vi "start.vi"(8 "error in (no error)":errorcluster, 11 "Pixelfly in":refnum<class "PixelflySA.lvclass">) -> (0 "error out":errorcluster, 3 "Pixelfly out":refnum<class "PixelflySA.lvclass">)   [LabVIEW 2011, in "PixelflySA.lvclass"]
uses:
  PixelflySA.lvclass
  Tools/CameraSettings/PixelFlySettings/PixelflySettings.lvclass
  PixelflySA.lvclass/PixelflySA.ctl
  Channels.lvlib
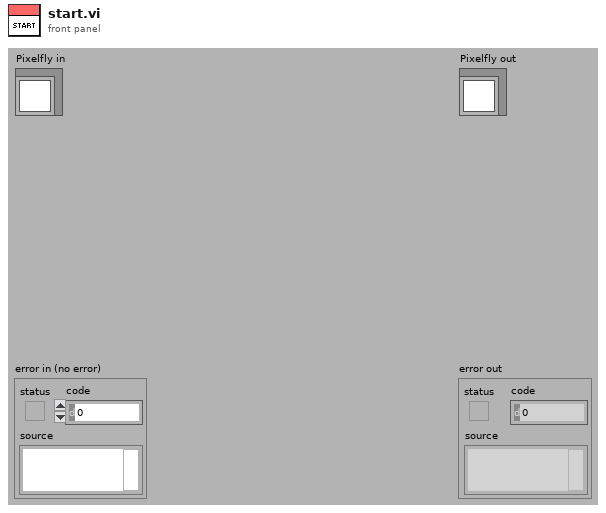
[diagram p1: front panel]
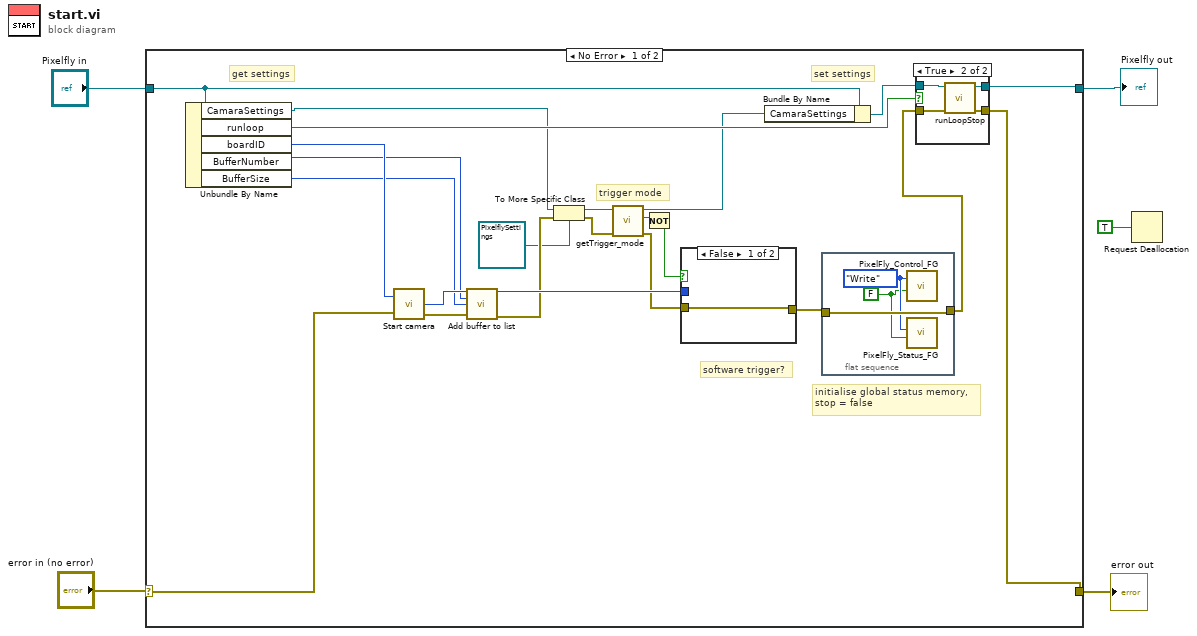
[diagram p0: block diagram]
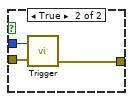
[diagram p3: hidden frame]
diagram:
  n1 = case shown="No Error" "error in (no error)" {
    selector: "error in (no error)" -> [w10 w42]
    tunnel: [w14 w42] -> w4
    tunnel: [w15 w43] -> w3
    tunnel: "Pixelfly in" -> [w9 w43]
    frame No Error {
      # "initialise global status memory,\nstop = false"
      # "set settings"
      # "get settings"
      # "trigger mode"
      # "software trigger?"
      n2 = Unbundle By Name(w9) -> ("CamaraSettings"=w11:refnum<class "CamaraSettings.lvclass">, "runloop"=w13:bool, "boardID"=w25:i32, "BufferNumber"=w24:i32, "BufferSize"=w23:i32)
      n3 = call <instrlib>:"Start camera.vi"("Handle in"=w25, "error in (no error)"=w10) -> ("Handle out"=w28:i32, "error out"=w27:errorcluster)  [unwired: 1 out]
      n4 = call <instrlib>:"Add buffer to list.vi"("Handle in"=w28, "Buffer in"=w24, "size"=w23, "error in (no error)"=w27) -> ("Handle out"=w26:i32, "error out"=w22:errorcluster)  [unwired: 9 in, 1 out]
      n5 = To More Specific Class(target class=refnum<class "PixelflySettings.lvclass"> refnum ("Tools.lvlib:Settings.lvlib:PixelflySettings.lvclass"), reference=w11, error in=w22) -> (specific class reference=w21:refnum<class "PixelflySettings.lvclass">, error out=w20:errorcluster)
      n6 = call "getTrigger_mode.vi"("error in (no error)"=w20, "PixelflySettings in"=w21) -> ("error out"=w18:errorcluster, "trigger_mode"=w17:bool, "PixelflySettings out"=w7:refnum<class "PixelflySettings.lvclass">)  [unwired: 7 in]
      n7 = Not(x=w17) -> (.not. x?=w16:bool)
      n8 = case shown="False" w16 {
        tunnel: w26 -> [_ w41]
        tunnel: w18 -> [w38 w40]
        tunnel: [w38 w39] -> w12
        frame False {
        }
        frame True {
          n9 = call <instrlib>:"Trigger.vi"("Handle in"=w41, "error in (no error)"=w40) -> ("error out"=w39:errorcluster)  [unwired: 2 out]
        }
      }
      n10 = Bundle By Name(cluster=w9, "CamaraSettings"=w7) -> (w8:refnum<class "PixelflySA.lvclass">)
      n11 = flat-sequence {
        tunnel: [w31] -> w6
        tunnel: w12 -> [w31]
        frame #0 {
          w30 = enum16{"Write", "Read"}."Write" ("Action")
          w29 = FALSE
          n12 = call "PixelFly_Control_FG.vi"("stop"=w29, "Action"=w30) -> ()  [unwired: 9 in, 1 out]
          n13 = call "PixelFly_Status_FG.vi"("stop"=w29, "Action"=w30) -> ()  [unwired: 9 in, 1 out]
        }
      }
      n14 = case shown="True" w13 {
        tunnel: [w33 w37] -> w15
        tunnel: [w32 w36] -> w14
        tunnel: w8 -> [w33 w35]
        tunnel: w6 -> [w32 w34]
        frame False {
        }
        frame True {
          n15 = call "runLoopStop.vi"("error in (no error)"=w34, "Pixelfly in"=w35) -> ("error out"=w36:errorcluster, "Pixelfly out"=w37:refnum<class "PixelflySA.lvclass">)  [unwired: 8 in]
        }
      }
    }
    frame Error {
    }
  }
  "error out" <- w4
  "Pixelfly out" <- w3
  n16 = Request Deallocation(TRUE ("flag")) -> ()
